vi "2013 FLL Scoring.vi"(11 "Array":cluster{"Name":string, "Value":string}[](array[cluster])) -> (0 "error out":errorcluster, 2 "Total Score":dbl)   [LabVIEW 2013]
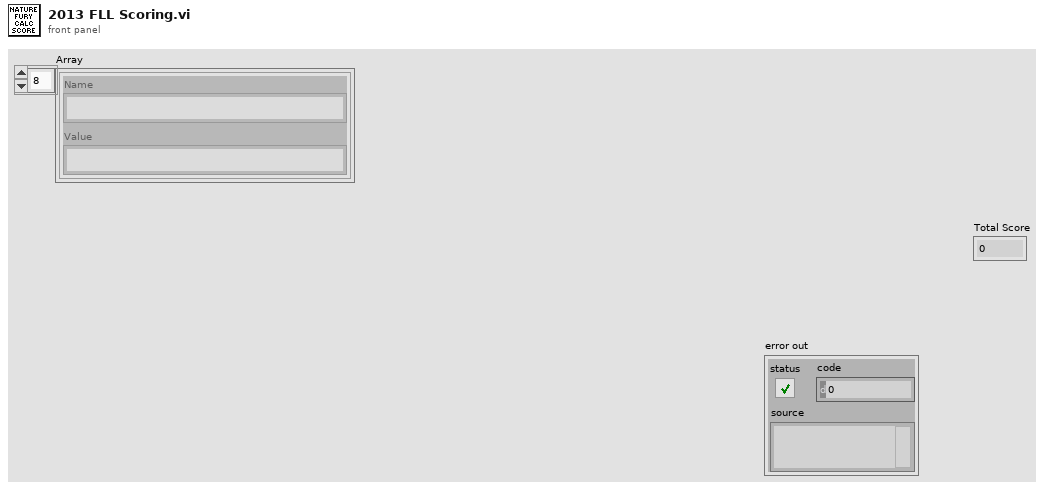
[diagram p1: front panel]
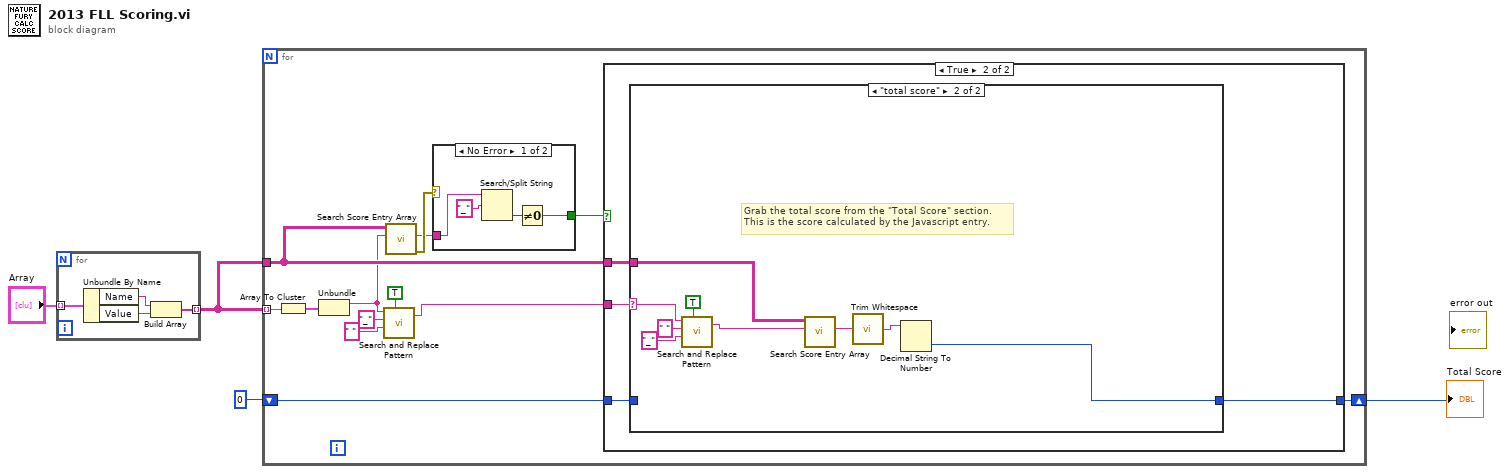
[diagram p0: block diagram]
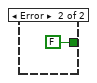
[diagram p4: hidden frame]
diagram:
  n1 = for {
    tunnel: "Array" -> [w8] mode=indexing
    tunnel: [w5] -> w1 mode=indexing
    n2 = Unbundle By Name(w8) -> ("Name"=w7:string, "Value"=w6:string)
    n3 = Build Array(w7, w6) -> (w5:string[])
  }
  n4 = for {
    shift-right: [w18] -> w2
    shift-left: 0 -> [w21]
    tunnel: w1 -> [w20] mode=indexing
    tunnel: w1 -> [w13]
    n5 = Array To Cluster(array=w20) -> (cluster=w19:cluster{"[0]":string, "[1]":string})
    n6 = Unbundle(w19) -> ("[0]"=w12:string)  [unwired: 1 out]
    n7 = call <vilib>:"Search and Replace Pattern.vi"("string"=w12, "regular expression (\"\")"="_" ("regular expression (\"\")"), "replace string (\"\")"=" " ("replace string (\"\")"), "replace all? (F)"=TRUE) -> ("result string"=w14:string)  [unwired: 1 in, 1 out]
    n8 = call "Search Score Entry Array.vi"("Item Name"=w12, "Array"=w13) -> ("error out"=w11:errorcluster, "Value"=w10:string)  [unwired: 6 in, 2 out]
    n9 = case shown="No Error" w11 {
      tunnel: w10 -> [w39 _]
      tunnel: [w37 FALSE] -> w9
      frame No Error {
        n10 = Search/Split String(string=w39, search string/char (-)="_") -> (offset of match=w38:i32)  [unwired: 1 in, 2 out]
        n11 = Not Equal To 0?(x=w38) -> (x != 0?=w37:bool)
      }
      frame Error {
      }
    }
    n12 = case shown="True" w9 {
      tunnel: w21 -> [w22 w26]
      tunnel: [w22 w25] -> w18
      tunnel: w14 -> [_ w24]
      tunnel: w13 -> [_ w23]
      frame False {
      }
      frame True {
        n13 = case shown="\"total score\"" w24 {
          selector: w24 -> [_ w36]
          tunnel: w26 -> [w27 _]
          tunnel: [w27 w28] -> w25
          tunnel: w23 -> [_ w32]
          frame "0", Default {
          }
          frame "total score" {
            # "Grab the total score from the \"Total Score\" section.\nThis is the score calculated by the Javascript entry."
            n14 = call <vilib>:"Search and Replace Pattern.vi"("string"=w36, "regular expression (\"\")"=" " ("regular expression (\"\")"), "replace string (\"\")"="_" ("replace string (\"\")"), "replace all? (F)"=TRUE) -> ("result string"=w31:string)  [unwired: 1 in, 1 out]
            n15 = call "Search Score Entry Array.vi"("Item Name"=w31, "Array"=w32) -> ("Value"=w29:string)  [unwired: 6 in, 3 out]
            n16 = call <vilib>:"Trim Whitespace.vi"("string"=w29) -> ("trimmed string"=w30:string)  [unwired: 1 in]
            n17 = Decimal String To Number(string=w30) -> (number=w28:i32)  [unwired: 2 in, 1 out]
          }
        }
      }
    }
  }
  "Total Score" <- w2
